vi "S2C_M2p5942_Poly_Channels.vi"(8 "Error In":errorcluster, 10 "Channels":T1={"CH3 Offset"=0, "CH3 Type"=0, "CH3 Term"=0, "CH3 Range"=2, "CH3 Enable"=TRUE, "CH2 Offset"=0, "CH2 Type"=0, "CH2 Term"=0, "CH2 Range"=2, "CH2 Enable"=TRUE, "CH1 Offset"=0, "CH1 Type"=0, "CH1 Term"=0, "CH1 Range"=2, "CH1 Enable"=TRUE, "CH0 Offset"=0, "CH0 Type"=0, "CH0 Term"=0, "CH0 Range"=2, "CH0 Enable"=TRUE} {"CH0 Range" items=["±200 mV", "±500 mV", "±1000 mV", "±2000 mV", "±5000 mV", "±10000 mV"]; "CH0 Term" items=["1 MOhm", "50 Ohm"]; "CH0 Type" items=["Single-ended", "Differential"]; "CH1 Range" items=["±200 mV", "±500 mV", "±1000 mV", "±2000 mV", "±5000 mV", "±10000 mV"]; "CH1 Term" items=["1 MOhm", "50 Ohm"]; "CH1 Type" items=["Single-ended", "Differential"]; "CH2 Range" items=["±200 mV", "±500 mV", "±1000 mV", "±2000 mV", "±5000 mV", "±10000 mV"]; "CH2 Term" items=["1 MOhm", "50 Ohm"]; "CH2 Type" items=["Single-ended", "Differential"]; "CH3 Range" items=["±200 mV", "±500 mV", "±1000 mV", "±2000 mV", "±5000 mV", "±10000 mV"]; "CH3 Term" items=["1 MOhm", "50 Ohm"]; "CH3 Type" items=["Single-ended", "Differential"]}, 11 "Settings":T2={"Driver"="M2p5942", "Command"="Channels", "Return"="ErrorStatus", "Parameters"="", "Timeout"=10.0}) -> (0 "Error Out":errorcluster, 3 "Response":string)   [LabVIEW 2015]
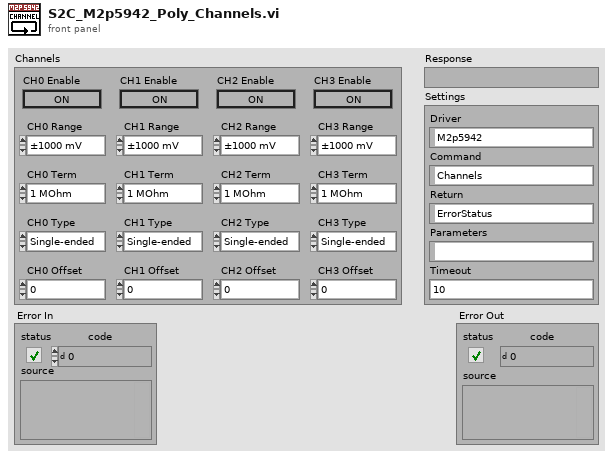
[diagram p1: front panel]
types:
  T1 = cluster{"CH3 Offset":i32, "CH3 Type":u16, "CH3 Term":u16, "CH3 Range":u16, "CH3 Enable":bool, "CH2 Offset":i32, "CH2 Type":u16, "CH2 Term":u16, "CH2 Range":u16, "CH2 Enable":bool, "CH1 Offset":i32, "CH1 Type":u16, "CH1 Term":u16, "CH1 Range":u16, "CH1 Enable":bool, "CH0 Offset":i32, "CH0 Type":u16, "CH0 Term":u16, "CH0 Range":u16, "CH0 Enable":bool}
  T2 = cluster{"Driver":string, "Command":string, "Return":string, "Parameters":string, "Timeout":dbl}
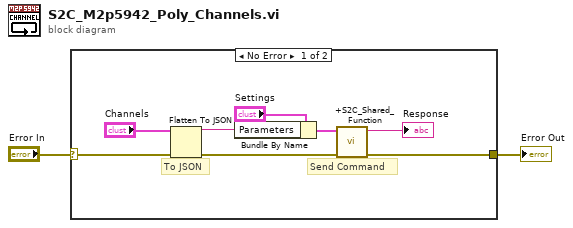
[diagram p0: block diagram]
diagram:
  n1 = case shown="No Error" "Error In" {
    selector: "Error In" -> [w6 w11]
    tunnel: [w5 w11] -> w1
    frame No Error {
      # "To JSON"
      # "Send Command"
      n2 = Flatten To JSON(anything="Channels", error in (no error)=w6) -> (JSON string=w7:string, 11:w9:errorcluster)  [unwired: 1 in]
      n3 = Bundle By Name(cluster="Settings", "Parameters"=w7) -> (w10:T2)
      n4 = call "+S2C_Shared_Function.vi"("Error In"=w9, "Settings"=w10) -> ("Error Out"=w5:errorcluster, "Response"=→"Response":string)  [unwired: 8 in]
    }
    frame Error {
    }
  }
  "Error Out" <- w1
